vi "Start_Sweep_Manual_text.vi"(8 "Rate":dbl, 11 "Setpoint":dbl) -> ()   [LabVIEW 2016]
uses:
  Instrument_Setup.vi
panel:
  in  "Rate 2":dbl
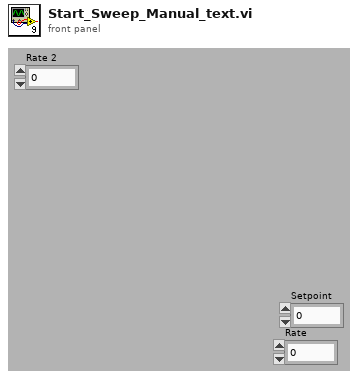
[diagram p1: front panel]
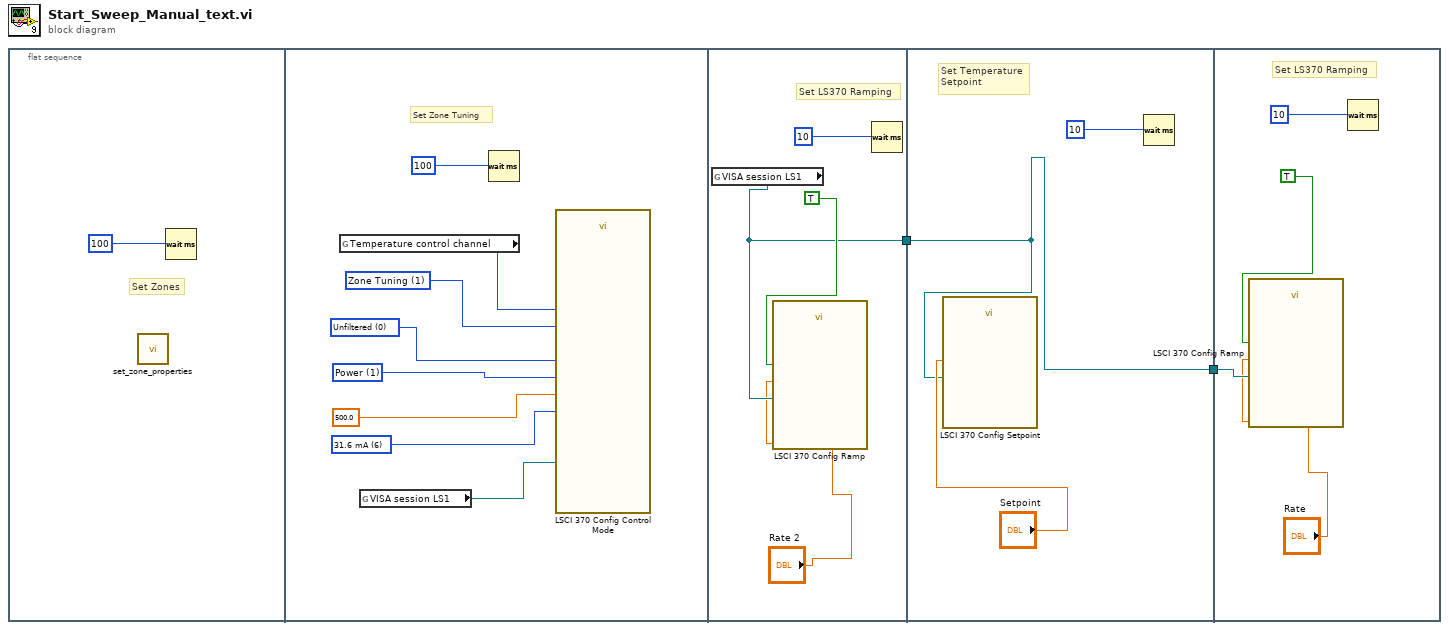
[diagram p0: block diagram]
diagram:
  n1 = flat-sequence {
    tunnel: [w13] -> w1
    tunnel: [w16] -> w2
    tunnel: w1 -> [w16]
    tunnel: w2 -> [w21]
    frame #0 {
      # "Set Zones"
      n2 = call "set_zone_properties.vi"() -> ()  [unwired: 1 in]
      n3 = Wait (ms)(milliseconds to wait=100) -> ()  [unwired: 1 out]
    }
    frame #1 {
      w10 = u16 6 items=["31.6 uA", "100 uA", "316 uA", "1.00 mA", "3.16 mA", "10.0 mA", "31.6 mA", "100 mA"] ("Maximum Heater Range (0: 31.6 uA)")
      w8 = u16 1 items=["Current", "Power"] ("Heater Output Display (0: Current)")
      w7 = u16 0 items=["Unfiltered", "Filtered"] ("Filtered Readings (0: Unfiltered)")
      w6 = u16 1 items=["Closed Loop PID", "Zone Tuning", "Open Loop", "Off"] ("Control Mode (0: Closed Loop PID)")
      # "Set Zone Tuning"
      n4 = global read "Instrument_Setup.vi" "Temperature control channel"() -> (w5:i32)
      n5 = global read "Instrument_Setup.vi" "VISA session LS1"() -> (w11:refnum<visa-resource-name>)
      n6 = Wait (ms)(milliseconds to wait=100) -> ()  [unwired: 1 out]
      n7 = call "LSCI 370 Config Control Mode.vi"("VISA session"=w11, "Control Mode (0: Closed Loop PID)"=w6, "Channel (1)"=w5, "Filtered Readings (0: Unfiltered)"=w7, "Heater Output Display (0: Current)"=w8, "Heater Resistance (100.00)"=500.0, "Maximum Heater Range (0: 31.6 uA)"=w10) -> ()  [unwired: 7 in, 2 out]
    }
    frame #2 {
      # "Set LS370 Ramping"
      n8 = global read "Instrument_Setup.vi" "VISA session LS1"() -> (w13:refnum<visa-resource-name>)
      n9 = call "LSCI 370 Config Ramp.vi"("VISA session"=w13, "Rate Value (0.001)"="Rate 2", "Ramping On/Off (F: Ramping Off)"=TRUE) -> ()  [unwired: 11 in, 2 out]
      n10 = Wait (ms)(milliseconds to wait=10) -> ()  [unwired: 1 out]
    }
    frame #3 {
      # "Set Temperature\nSetpoint"
      n11 = call "LSCI 370 Config Setpoint.vi"("VISA session"=w16, "Setpoint (0.00000E+0)"="Setpoint") -> ()  [unwired: 12 in, 2 out]
      n12 = Wait (ms)(milliseconds to wait=10) -> ()  [unwired: 1 out]
    }
    frame #4 {
      # "Set LS370 Ramping"
      n13 = call "LSCI 370 Config Ramp.vi"("VISA session"=w21, "Rate Value (0.001)"="Rate", "Ramping On/Off (F: Ramping Off)"=TRUE) -> ()  [unwired: 11 in, 2 out]
      n14 = Wait (ms)(milliseconds to wait=10) -> ()  [unwired: 1 out]
    }
  }
